vi "Initialize From Config.vi"(8 "error in":errorcluster, 9 "Modules":refnum<class "TBM module execution interface.lvclass">[](array[class]), 10 "Module Configurations":refnum<class "TBM module configuration.lvclass">[](array[class]), 11 "Engine Configuration":refnum<class "Standard Engine Configuration.lvclass">) -> (0 "error out":errorcluster, 3 "Engine Data Out":T1={"timed loop timer source"={"Processor"=-2, "Priority"=0, "timing source dt"=2, "timer source"=refnum}, "control loop data"={"engine tag bus"={"Double"=[], "Single"=[], "I64"=[], "I32"=[], "I16"=[], "I8"=[], "U64"=[], "U32"=[], "U16"=[], "U8"=[], "Boolean"=[], "String"=[], "Array of Double"=[], "Array of Single"=[], "Array of I64"=[], "Array of I32"=[], "Array of I16"=[], "Array of I8"=[], "Array of U64"=[], "Array of U32"=[], "Array of U16"=[], "Array of U8"=[], "Array of Boolean"=[], "Array of String"=[]}, "engine schedule"={"module run flags"=[], "decimation schedule"={"decimations"=[], "offsets"=[]}}, "module information"=[]}, "status reporting"={"late? index (bool)"=-1, "late count index (U32)"=-1, "dt (ns) index (U64)"=-1, "execution time (ns) index (U64)"=-1}})   [LabVIEW 2013, in "Standard Engine Runtime.lvclass"]
doc: "This VI contains all of the logic necessary for configuring the engine based on a given engine configuration, and an array of modules with their configurations. \n\nFirst it allows the modules to finish configuring themselves by calling their dynamic configuration and mapping functions. \n\nThen it calls the Init method for each module and initializes their channel data space as well as the engine's tag data space. \n\nIt also initializes all of the other features of the engine including the timing source, decimation, error handling, execution order, etc."
uses:
  Standard Engine Runtime.lvclass
  main engine/Engine Data.ctl
  <vilib>/NI/Module Timing Source/timing source/TBM timing source.lvclass
  main engine/timed loop timing sources.ctl
  main engine/control loop data.ctl
  <vilib>/NI/Tag Bus/table/data table.ctl
  main engine/engine run schedule.ctl
  main engine/engine decimation schedule.ctl
  main engine/full module data.ctl
  <vilib>/NI/Tag Bus Module Framework/runtime/TBM module execution interface.lvclass
  main engine/module run state.ctl
  async executor/asynchronous executor reference.ctl
  async executor/async message to executor.ctl
  async command notification.ctl
  async error info.ctl
  <vilib>/NI/Tag Bus Module Framework/runtime/error classification.ctl
  <vilib>/NI/Tag Bus Module Framework/module configuration/TBM module configuration.lvclass
  main engine/module method data.ctl
  <vilib>/NI/Tag Bus/table/transfer specification.ctl
  <vilib>/NI/Tag Bus/tag/Data Type.ctl
  main engine/fault handling spec.ctl
  Configuration/Error Actions.ctl
  main engine/status reporting data.ctl
  Configuration/Standard Engine Configuration.lvclass
  Configuration/Standard Engine Configuration.lvclass/Standard Engine Configuration.ctl
  <vilib>/NI/Configuration Framework/serializable configuration/NISE_CEF_serializable configuration.lvclass/NISE_CEF_serializable configuration.ctl
  <vilib>/NI/Module Timing Source/standard timing source/ms timing source.lvclass
  <vilib>/NI/Module Timing Source/usec timing source/usec timing source.lvclass
  <vilib>/NI/Module Timing Source/scan engine timing source/scan engine timing source.lvclass
  <vilib>/NI/Module Execution Interface/Engine Configuration/engine configuration.lvclass/engine configuration.ctl
  <vilib>/NI/Tag Bus/dictionary/data dictionary.lvclass/data dictionary.ctl
  <vilib>/NI/Tag Bus/dictionary/lookup polymorphs/locate double.vi
  <vilib>/NI/Tag Bus/dictionary/lookup polymorphs/locate I32.vi
  Configuration/Read Processor.vi
  Configuration/Read Priority.vi
  Configuration/Read Master Timing Module.vi
  Configuration/Read Timing Source Type.vi
  Configuration/Read enable module timing info.vi
  <vilib>/NI/Tag Bus/dictionary/search/find data index.vi
  <vilib>/NI/Tag Bus/dictionary/search/search string list.vi
  Configuration/Read Timing Source dt.vi
  <vilib>/Utility/LVClass/Get LV Class Name.vi
  <vilib>/NI/Configuration Framework/error generator/NISE_error generator.vi
  Configuration/Find Module Specific Config.vi
  <vilib>/NI/Configuration Framework/serializable configuration/get alias.vi
  <vilib>/NI/Tag Bus/dictionary/tag not found.vi
  <vilib>/Utility/RT CPU pool selections.ctl
  <vilib>/NI/Tag Bus/dictionary/data dictionary.lvclass
  <vilib>/NI/Module Execution Interface/Engine Configuration/engine configuration.lvclass
  <vilib>/NI/Module Execution Interface/Engine Runtime/Engine Runtime Interface.lvclass
  main engine/main engine.lvlib
  <vilib>/NI/Configuration Framework/serializable configuration/NISE_CEF_serializable configuration.lvclass
  <vilib>/NI/Tag Bus/table/data table.lvlib
  <vilib>/NI/Tag Bus/tag/tag descriptor.lvclass
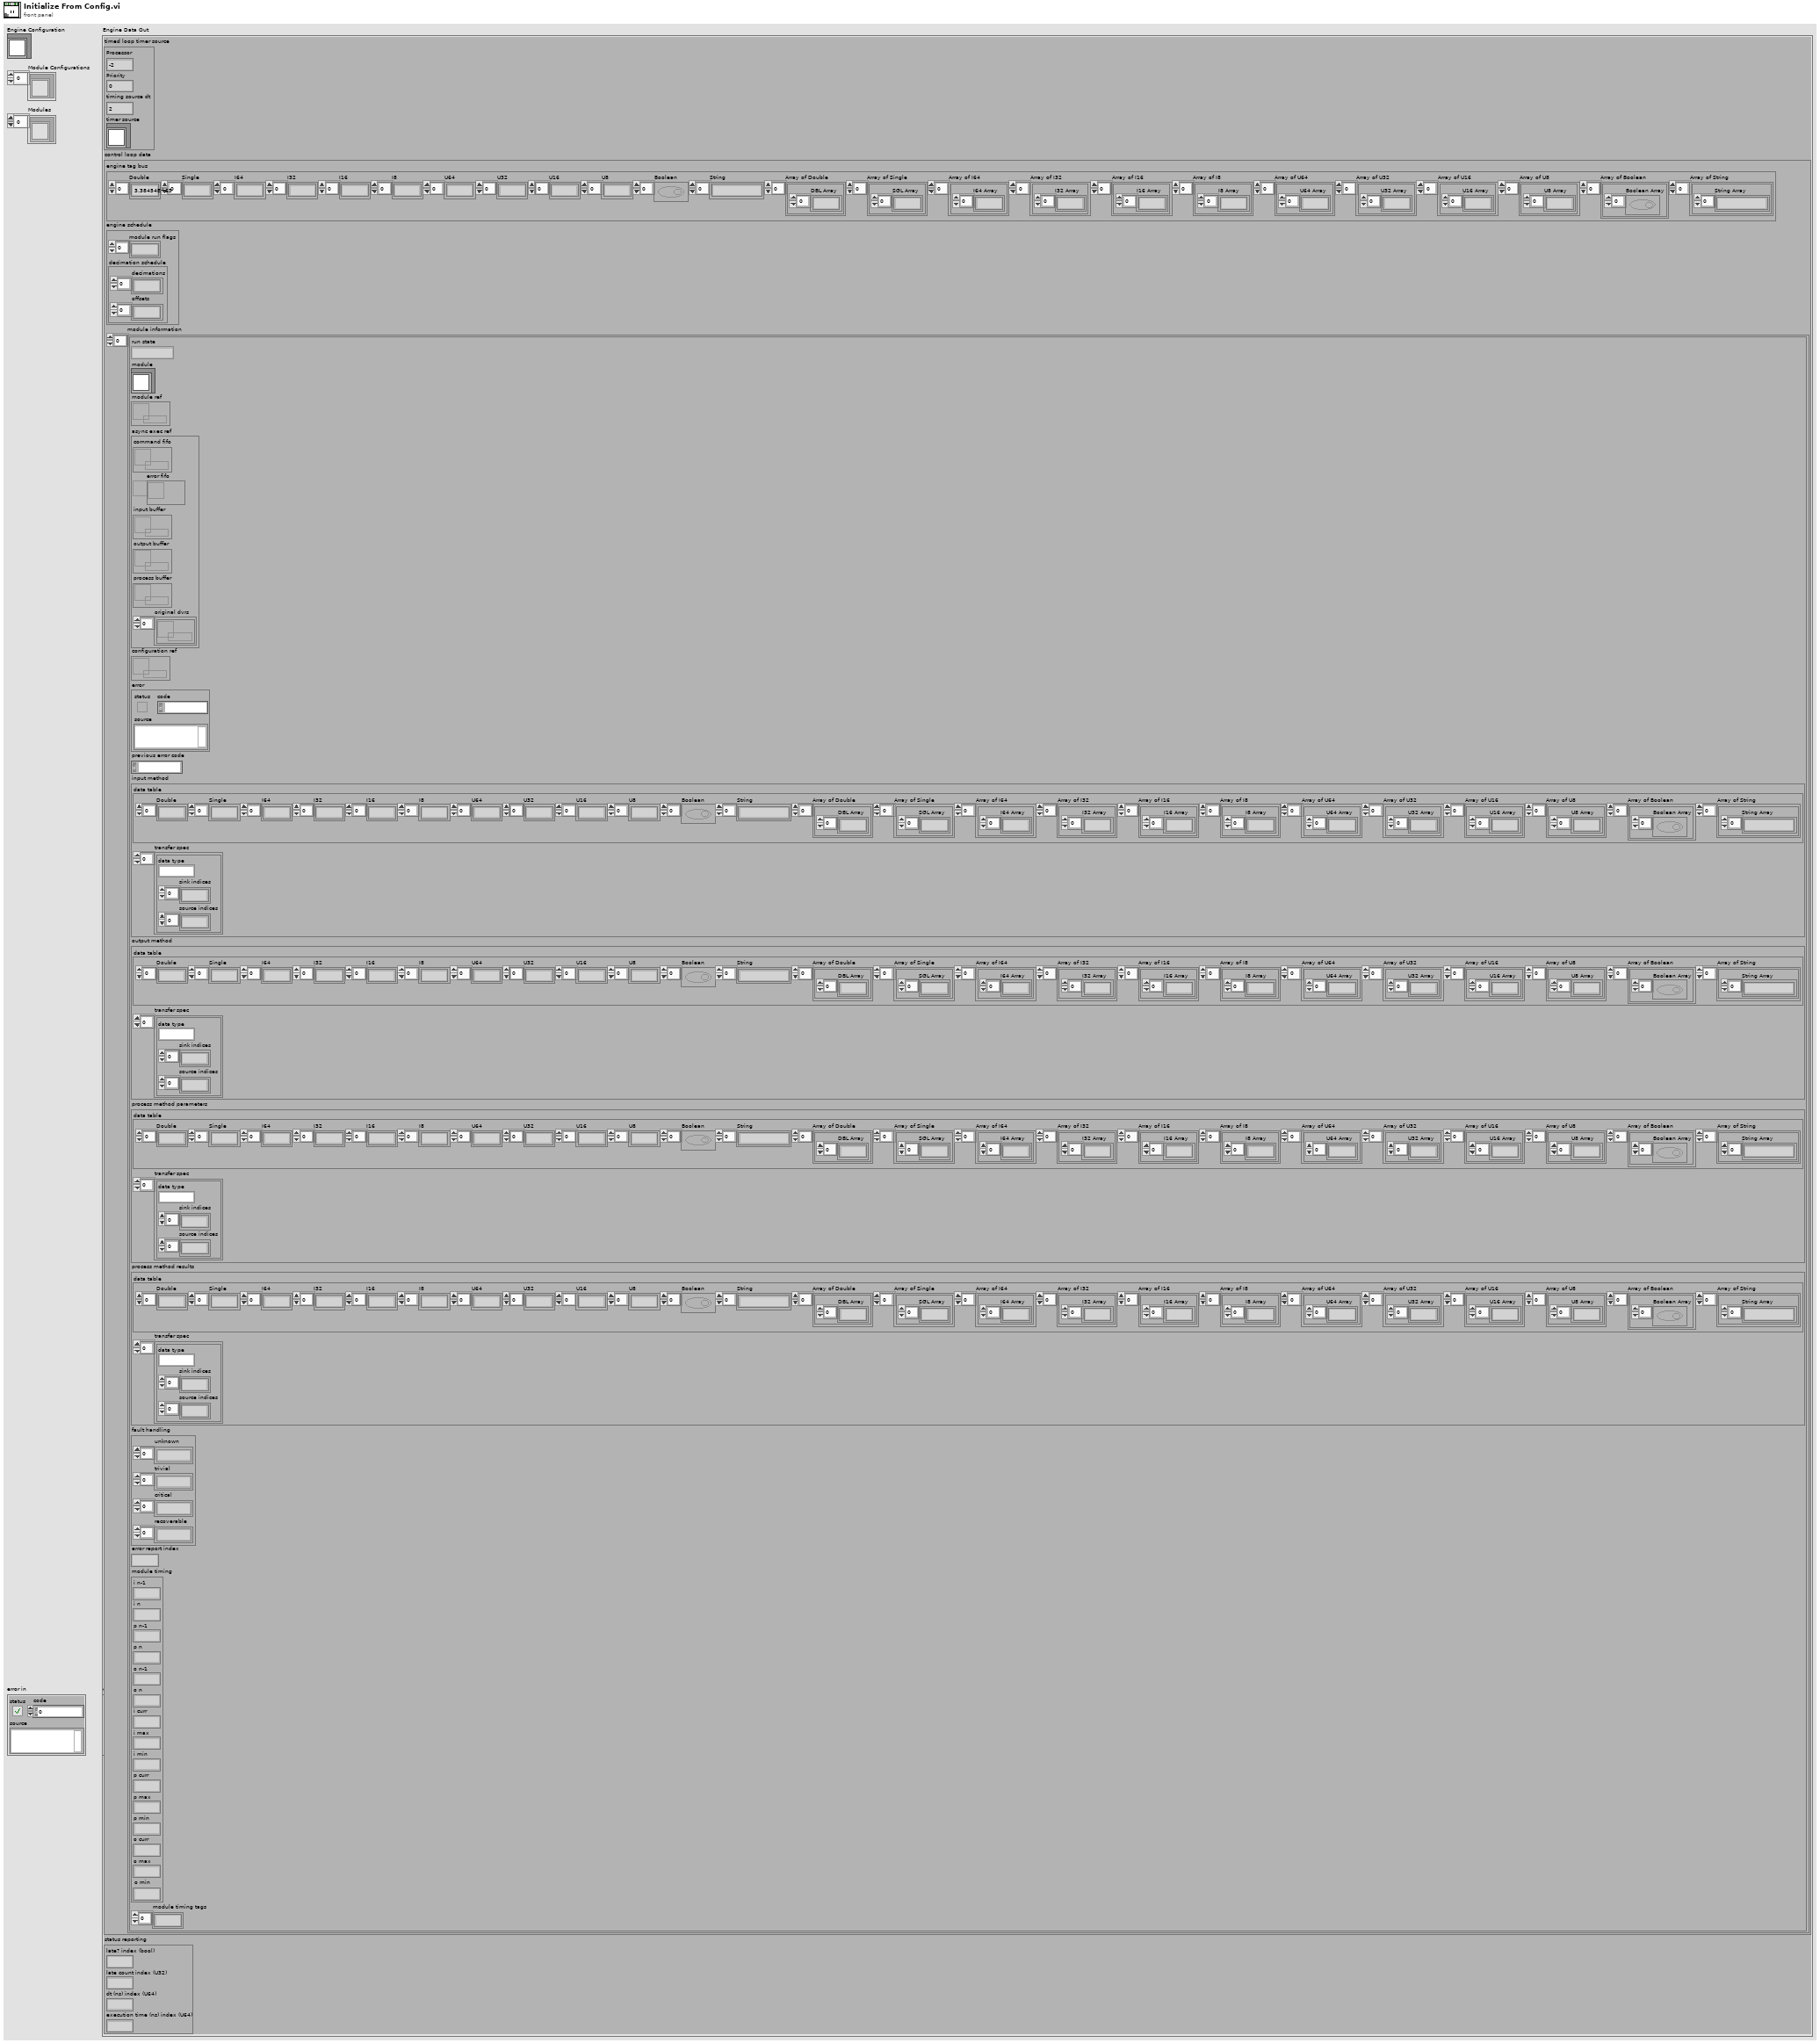
[diagram p1: front panel]
types:
  T1 = typedef "main engine.lvlib/Engine Data.ctl" = cluster{"timed loop timer source":T2, "control loop data":T3, "status reporting":T15}
  T2 = typedef "main engine.lvlib/timed loop timing sources.ctl" = cluster{"Processor":i32, "Priority":i32, "timing source dt":u32, "timer source":refnum<class "TBM timing source.lvclass">}
  T3 = typedef "main engine.lvlib/control loop data.ctl" = cluster{"engine tag bus":T4, "engine schedule":T5, "module information":T7[]}
  T4 = typedef "tag bus.lvlib/data table.lvlib/data table.ctl" = cluster{"Double":dbl[], "Single":sgl[], "I64":i64[], "I32":i32[], "I16":i16[], "I8":i8[], "U64":u64[], "U32":u32[], "U16":u16[], "U8":u8[], "Boolean":bool[], "String":string[], "Array of Double":cluster{"DBL Array":dbl[]}[], "Array of Single":cluster{"SGL Array":sgl[]}[], "Array of I64":cluster{"I64 Array":i64[]}[], "Array of I32":cluster{"I32 Array":i32[]}[], "Array of I16":cluster{"I16 Array":i16[]}[], "Array of I8":cluster{"I8 Array":i8[]}[], "Array of U64":cluster{"U64 Array":u64[]}[], "Array of U32":cluster{"U32 Array":u32[]}[], "Array of U16":cluster{"U16 Array":u16[]}[], "Array of U8":cluster{"U8 Array":u8[]}[], "Array of Boolean":cluster{"Boolean Array":bool[]}[], "Array of String":cluster{"String Array":string[]}[]}
  T5 = typedef "main engine.lvlib/engine run schedule.ctl" = cluster{"module run flags":u8[], "decimation schedule":T6}
  T6 = typedef "main engine.lvlib/engine decimation schedule.ctl" = cluster{"decimations":u16[], "offsets":u16[]}
  T7 = typedef "main engine.lvlib/full module data.ctl" = cluster{"run state":T8, "module":refnum<class "TBM module execution interface.lvclass">, "module ref":refnum<data-value>, "async exec ref":T9, "configuration ref":refnum<data-value>, "error":errorcluster, "previous error code":i32, "input method":T10, "output method":T10, "process method parameters":T10, "process method results":T10, "fault handling":T13, "error report index ":i32, "module timing":cluster{"i n-1":dbl, "i n":dbl, "p n-1":dbl, "p n":dbl, "o n-1":dbl, "o n":dbl, "i curr":dbl, "i max":dbl, "i min":dbl, "p curr":dbl, "p max":dbl, "p min":dbl, "o curr":dbl, "o max":dbl, "o min":dbl}, "module timing tags":i32[]}
  T8 = typedef "main engine.lvlib/module run state.ctl" = enum16{"sync", "async"}
  T9 = typedef "main engine.lvlib/asynchronous executor reference.ctl" = cluster{"command fifo":refnum<k33>, "error fifo":refnum<k33>, "input buffer":refnum<k33>, "output buffer":refnum<k33>, "process buffer":refnum<k33>, "original dvrs":refnum<data-value>[]}
  T10 = typedef "main engine.lvlib/module method data.ctl" = cluster{"data table":T4, "transfer spec":T11[]}
  T11 = typedef "tag bus.lvlib/data table.lvlib/transfer specification.ctl" = cluster{"data type":T12, "sink indices":i32[], "source indices":i32[]}
  T12 = typedef "tag bus.lvlib/tag descriptor.lvclass/Data Type.ctl" = enum16{"Double", "Single", "I64", "I32", "I16", "I8", "U64", "U32", "U16", "U8", "Boolean", "String", "Array of Double", "Array of Single", "Array of I64", "Array of I32", "Array of I16", "Array of I8", "Array of U64", "Array of U32", "Array of U16", "Array of U8", "Array of Boolean", "Array of String"}
  T13 = typedef "main engine.lvlib/fault handling spec.ctl" = cluster{"unknown":T14[], "trivial":T14[], "critical":T14[], "recoverable":T14[]}
  T14 = typedef "Standard Engine Configuration.lvclass/Error Actions.ctl" = enum16{"Clear", "Notify", "Stop Component", "Stop Engine", "Safe State", "Attempt Recovery"}
  T15 = typedef "main engine.lvlib/status reporting data.ctl" = cluster{"late? index (bool)":i32, "late count index (U32)":i32, "dt (ns) index (U64)":i32, "execution time (ns) index (U64)":i32}
  T16 = typedef "Standard Engine Configuration.lvclass/Supported Timing Sources.ctl" = enum16{"Use Module Timing Source", "1 kHz Clock", "1 MHz Clock", "Synchronize to Scan Engine"}
  T17 = cluster{"execution order priority":i32, "Component Runtime Interface.lvclass":refnum<class "TBM module execution interface.lvclass">, "configuration out":refnum<class "TBM module configuration.lvclass">}
  T18 = cluster{"execution order priority":i32, "Component Runtime Interface.lvclass":refnum<class "TBM module execution interface.lvclass">, "configuration out":refnum<class "TBM module configuration.lvclass">}[]
  T19 = typedef "TBM channel.lvclass/data tables.ctl" = cluster{"input data":T20, "processing parameter":T20, "processing result":T20, "output data":T20}
  T20 = typedef "tag bus.lvlib/dictionary table pair.ctl" = cluster{"data dictionary":refnum<class "data dictionary.lvclass">, "data table":T4}
  T21 = typedef "TBM module execution interface.lvclass/execution settings.ctl" = cluster{"reads inputs":bool, "processes data":bool, "writes outputs":bool}
  T22 = typedef "Standard Engine Configuration.lvclass/error responses.ctl" = cluster{"unknown":T23, "trivial":T23, "critical":T23, "recoverable":T23}
  T23 = typedef "Standard Engine Configuration.lvclass/error options.ctl" = cluster{"clear":bool, "notify":bool, "remove module":bool, "abort engine":bool, "go to safe state":bool, "recover module":bool}
  T24 = typedef "Standard Engine Configuration.lvclass/Module Decimation.ctl" = cluster{"Decimation":u16, "Offset":u16, "sort order":i32, "async?":bool}
  T25 = typedef "Standard Engine Configuration.lvclass/timing reporting tags.ctl" = cluster{"late index (bool)":string, "late count index (U32)":string, "current dt ns(U64)":string, "last exec time ns(U64)":string}
  T26 = typedef "NI_Real-Time Target Support.lvlib/RT CPU pool selections.ctl" = enum16{"System & Timed Structures", "System", "Timed Structures", "Reserved"}
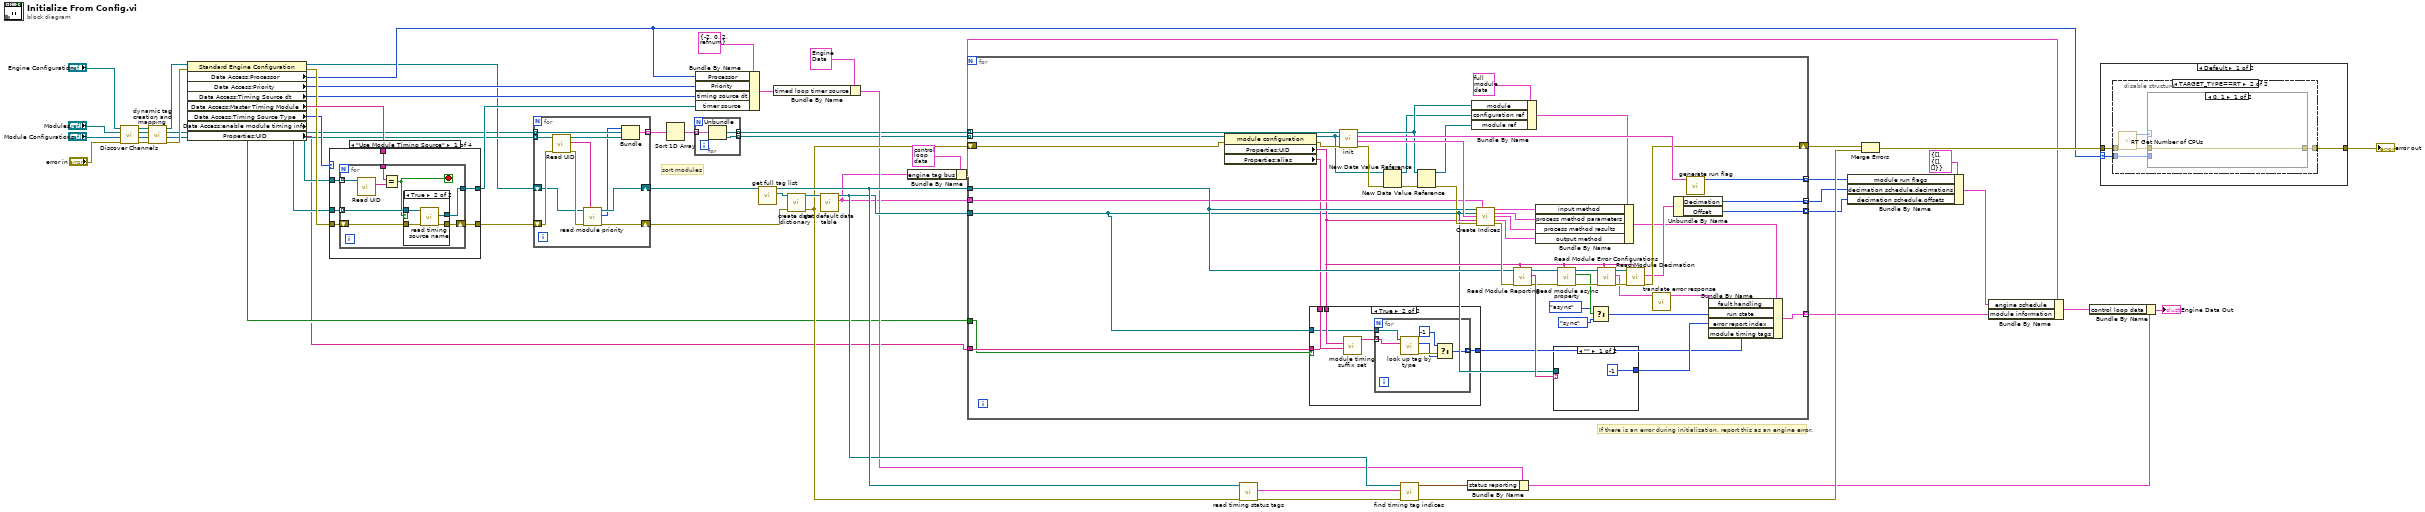
[diagram p0: block diagram]
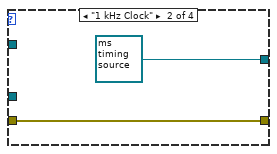
[diagram p3: hidden frame]
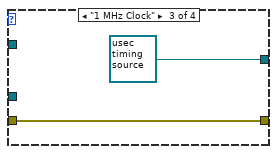
[diagram p4: hidden frame]
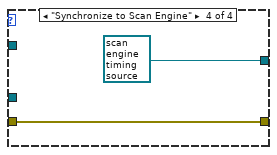
[diagram p5: hidden frame]
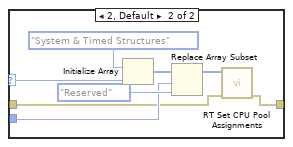
[diagram p7: hidden frame]
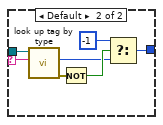
[diagram p10: hidden frame]
diagram:
  # "sort modules"
  # "If there is an error during initialization, report this as an engine error."
  n1 = call <vilib>:"Discover Channels.vi"("error in (no error)"="error in", "module configurations"="Module Configurations", "modules"="Modules", "engine configuration"="Engine Configuration") -> ("error out"=w52:errorcluster, "module configurations out"=w53:refnum<class "TBM module configuration.lvclass">[], "modules out"=w54:refnum<class "TBM module execution interface.lvclass">[], "engine configuration out"=w55:refnum<class "Standard Engine Configuration.lvclass">)  [unwired: 4 in]
  n2 = call <vilib>:"dynamic tag creation and mapping.vi"("error in"=w52, "module configurations"=w53, "modules"=w54, "engine configuration in"=w55) -> ("error out"=w46:errorcluster, "module configurations out"=w17:refnum<class "TBM module configuration.lvclass">[], "modules out"=w14:refnum<class "TBM module execution interface.lvclass">[], "engine configuration out"=w47:refnum<class "Standard Engine Configuration.lvclass">)  [unwired: 4 in]
  n3 = property class="Standard Engine Configuration"(reference=w47, error in=w46) -> (reference out=w16:refnum<class "Standard Engine Configuration.lvclass">, error out=w41:errorcluster, "Data Access:Processor"=w31:i32, "Data Access:Priority"=w30:i32, "Data Access:Timing Source dt"=w29:u32, "Data Access:Master Timing Module"=w42:string, "Data Access:Timing Source Type"=w32:T16, "Data Access:enable module timing info"=w2:bool, "Properties:UID"=w1:string)
  n4 = case shown="\"Use Module Timing Source\"" w32 {
    tunnel: [w60 refnum<class "ms timing source.lvclass"> refnum ("ms timing source.lvclass") refnum<class "usec timing source.lvclass"> refnum ("usec timing source.lvclass") refnum<class "scan engine timing source.lvclass"> refnum ("scan engine timing source.lvclass")] -> w40
    tunnel: w17 -> [w63 _ _ _]
    tunnel: w14 -> [w62 _ _ _]
    tunnel: w42 -> [w61 _ _ _]
    tunnel: [w59 w77 w79 w81] -> w13
    tunnel: w41 -> [w58 w77 w79 w81]
    frame "Use Module Timing Source" {
      n5 = for {
        tunnel: w63 -> [w71] mode=indexing
        tunnel: w62 -> [w68] mode=indexing
        tunnel: w61 -> [w69]
        tunnel: [w66] -> w60
        shift-right: [w65] -> w59
        shift-left: w58 -> [w64]
        stop <- w67 stop-if-true
        n6 = call <vilib>:"Read UID.vi"("configuration in"=w71) -> ("instance id"=w70:string)  [unwired: 8 in, 2 out]
        n7 = Equal?(x=w69, y=w70) -> (x = y?=w67:bool)
        n8 = case shown="True" w67 {
          tunnel: w68 -> [_ w76]
          tunnel: [_ w75] -> w66
          tunnel: [w72 w74] -> w65
          tunnel: w64 -> [w72 w73]
          frame False {
          }
          frame True {
            n9 = call-dynamic "read timing source name.vi"("error in"=w73, "module in"=w76) -> ("error out"=w74:errorcluster, "timing source"=w75:refnum<class "TBM timing source.lvclass">)  [unwired: 7 in, 1 out]
          }
        }
      }
    }
    frame "1 kHz Clock" {
    }
    frame "1 MHz Clock" {
    }
    frame "Synchronize to Scan Engine" {
    }
  }
  n10 = for {
    tunnel: w17 -> [w93] mode=indexing
    shift-right: [w89] -> w15
    shift-left: w16 -> [w87]
    tunnel: w14 -> [w86] mode=indexing
    shift-right: [w92] -> w12
    shift-left: w13 -> [w91]
    tunnel: [w83] -> w11 mode=indexing
    n11 = call <vilib>:"Read UID.vi"("error in"=w91, "configuration in"=w93) -> ("error out"=w90:errorcluster, "instance id"=w88:string, "configuration out"=w85:refnum<class "TBM module configuration.lvclass">)  [unwired: 7 in]
    n12 = call "read module priority.vi"("Module ID"=w88, "error in"=w90, "Standard Engine Repo Data in"=w87) -> ("error out"=w92:errorcluster, "execution order priority"=w84:i32, "Standard Engine Repo Data out"=w89:refnum<class "Standard Engine Configuration.lvclass">)  [unwired: 6 in]
    n13 = Bundle("execution order priority"=w84, "Component Runtime Interface.lvclass"=w86, "configuration out"=w85) -> (w83:T17)  [unwired: 1 in]
  }
  n14 = Sort 1D Array(array=w11) -> (sorted array=w10:T18)
  n15 = for {
    tunnel: w10 -> [w96] mode=indexing
    tunnel: [w95] -> w9 mode=indexing
    tunnel: [w94] -> w8 mode=indexing
    n16 = Unbundle(w96) -> ("Component Runtime Interface.lvclass"=w95:refnum<class "TBM module execution interface.lvclass">, "configuration out"=w94:refnum<class "TBM module configuration.lvclass">)  [unwired: 1 out]
  }
  n17 = Bundle By Name(cluster=T2 {"Processor"=-2, "Priority"=0, "timing source dt"=2, "timer source"=refnum} ("timed loop timer source"), "Processor"=w31, "Priority"=w30, "timing source dt"=w29, "timer source"=w40) -> (w27:T2)
  n18 = call <vilib>:"get full tag list.vi"("engine configuration in"=w15) -> ("tag list"=w45:refnum<class "tag descriptor.lvclass">[], "engine configuration out"=w39:refnum<class "Standard Engine Configuration.lvclass">)  [unwired: 9 in]
  n19 = Bundle By Name(cluster=T1 {"timed loop timer source"={"Processor"=-2, "Priority"=0, "timing source dt"=2, "timer source"=refnum}, "control loop data"={"engine tag bus"={"Double"=[], "Single"=[], "I64"=[], "I32"=[], "I16"=[], "I8"=[], "U64"=[], "U32"=[], "U16"=[], "U8"=[], "Boolean"=[], "String"=[], "Array of Double"=[], "Array of Single"=[], "Array of I64"=[], "Array of I32"=[], "Array of I16"=[], "Array of I8"=[], "Array of U64"=[], "Array of U32"=[], "Array of U16"=[], "Array of U8"=[], "Array of Boolean"=[], "Array of String"=[]}, "engine schedule"={"module run flags"=[], "decimation schedule"={"decimations"=[], "offsets"=[]}}, "module information"=[]}, "status reporting"={"late? index (bool)"=-1, "late count index (U32)"=-1, "dt (ns) index (U64)"=-1, "execution time (ns) index (U64)"=0}} ("Engine Data Out"), "timed loop timer source"=w27) -> (w26:T1)
  n20 = call <vilib>:"create data dictionary.vi"("error in"=w12, "system tags"=w45) -> ("error out"=w38:errorcluster, "data dictionary"=w44:refnum<class "data dictionary.lvclass">)  [unwired: 8 in]
  n21 = call <vilib>:"get default data table.vi"("data dictionary in"=w44) -> ("default data table"=w3:T4, "data dictionary out"=w35:refnum<class "data dictionary.lvclass">)  [unwired: 9 in]
  n22 = Bundle By Name(cluster=T3 {"engine tag bus"={"Double"=[], "Single"=[], "I64"=[], "I32"=[], "I16"=[], "I8"=[], "U64"=[], "U32"=[], "U16"=[], "U8"=[], "Boolean"=[], "String"=[], "Array of Double"=[], "Array of Single"=[], "Array of I64"=[], "Array of I32"=[], "Array of I16"=[], "Array of I8"=[], "Array of U64"=[], "Array of U32"=[], "Array of U16"=[], "Array of U8"=[], "Array of Boolean"=[], "Array of String"=[]}, "engine schedule"={"module run flags"=[], "decimation schedule"={"decimations"=[], "offsets"=[]}}, "module information"=[]} ("control loop data"), "engine tag bus"=w3) -> (w21:T3)
  n23 = for {
    tunnel: w8 -> [w141] mode=indexing
    shift-right: [w137] -> w57
    shift-left: w38 -> [w140]
    tunnel: w9 -> [w145] mode=indexing
    tunnel: w35 -> [w99]
    tunnel: w39 -> [w133]
    tunnel: [w132] -> w7 mode=indexing
    tunnel: [w130] -> w6 mode=indexing
    tunnel: [w129] -> w5 mode=indexing
    tunnel: [w111] -> w4 mode=indexing
    tunnel: w3 -> [w103]
    tunnel: w2 -> [w97]
    tunnel: w1 -> [w100]
    n24 = property class="module configuration"(reference=w141, error in=w140) -> (reference out=w118:refnum<class "TBM module configuration.lvclass">, error out=w136:errorcluster, "Properties:UID"=w101:string, "Properties:alias"=w102:string)
    n25 = case shown="True" w97 {
      tunnel: w102 -> [_ w151]
      tunnel: w101 -> [_ w150]
      tunnel: w100 -> [_ w149]
      tunnel: w99 -> [_ w148]
      tunnel: [_ w146] -> w98
      frame False {
      }
      frame True {
        n26 = call "module timing suffix set.vi"("mod alias"=w151, "mod id"=w150, "eng id"=w149) -> ("names"=w147:string[])  [unwired: 8 in]
        n27 = for {
          tunnel: w148 -> [w157]
          tunnel: w147 -> [w156] mode=indexing
          tunnel: [w152] -> w146 mode=indexing
          n28 = call-poly <vilib>:"look up tag by type.vi"("name"=w156, "data dictionary in"=w157) -> ("error out"=w155:errorcluster, "index"=w154:i32)  [unwired: 7 in, 1 out]
          n29 = Select(t=-1, s=w155, f=w154) -> (s? t:f=w152:i32)
        }
      }
    }
    n30 = call-dynamic "init.vi"("error in"=w136, "module configuration"=w118, "module in"=w145) -> ("error out"=w144:errorcluster, "data allocations"=w142:T19, "execution settings"=w143:T21, "module out"=w116:refnum<class "TBM module execution interface.lvclass">)  [unwired: 5 in]
    n31 = New Data Value Reference(data value=w118, error in=w144) -> (data value reference=w115:refnum<data-value>, error out=w120:errorcluster)
    n32 = New Data Value Reference(data value=w116, error in=w120) -> (data value reference=w117:refnum<data-value>, error out=w119:errorcluster)
    n33 = Bundle By Name(cluster=T7 {"run state"=enum."sync", "module"=refnum, "module ref"=refnum, "async exec ref"={"command fifo"=refnum, "error fifo"=refnum, "input buffer"=refnum, "output buffer"=refnum, "process buffer"=refnum, "original dvrs"=[]}, "configuration ref"=refnum, "error"={"status"=FALSE, "code"=0, "source"=""}, "previous error code"=0, "input method"={"data table"={"Double"=[], "Single"=[], "I64"=[], "I32"=[], "I16"=[], "I8"=[], "U64"=[], "U32"=[], "U16"=[], "U8"=[], "Boolean"=[], "String"=[], "Array of Double"=[], "Array of Single"=[], "Array of I64"=[], "Array of I32"=[], "Array of I16"=[], "Array of I8"=[], "Array of U64"=[], "Array of U32"=[], "Array of U16"=[], "Array of U8"=[], "Array of Boolean"=[], "Array of String"=[]}, "transfer spec"=[]}, "output method"={"data table"={"Double"=[], "Single"=[], "I64"=[], "I32"=[], "I16"=[], "I8"=[], "U64"=[], "U32"=[], "U16"=[], "U8"=[], "Boolean"=[], "String"=[], "Array of Double"=[], "Array of Single"=[], "Array of I64"=[], "Array of I32"=[], "Array of I16"=[], "Array of I8"=[], "Array of U64"=[], "Array of U32"=[], "Array of U16"=[], "Array of U8"=[], "Array of Boolean"=[], "Array of String"=[]}, "transfer spec"=[]}, "process method parameters"={"data table"={"Double"=[], "Single"=[], "I64"=[], "I32"=[], "I16"=[], "I8"=[], "U64"=[], "U32"=[], "U16"=[], "U8"=[], "Boolean"=[], "String"=[], "Array of Double"=[], "Array of Single"=[], "Array of I64"=[], "Array of I32"=[], "Array of I16"=[], "Array of I8"=[], "Array of U64"=[], "Array of U32"=[], "Array of U16"=[], "Array of U8"=[], "Array of Boolean"=[], "Array of String"=[]}, "transfer spec"=[]}, "process method results"={"data table"={"Double"=[], "Single"=[], "I64"=[], "I32"=[], "I16"=[], "I8"=[], "U64"=[], "U32"=[], "U16"=[], "U8"=[], "Boolean"=[], "String"=[], "Array of Double"=[], "Array of Single"=[], "Array of I64"=[], "Array of I32"=[], "Array of I16"=[], "Array of I8"=[], "Array of U64"=[], "Array of U32"=[], "Array of U16"=[], "Array of U8"=[], "Array of Boolean"=[], "Array of String"=[]}, "transfer spec"=[]}, "fault handling"={"unknown"=[], "trivial"=[], "critical"=[], "recoverable"=[]}, "error report index "=0, "module timing"={"i n-1"=0.0, "i n"=0.0, "p n-1"=0.0, "p n"=0.0, "o n-1"=0.0, "o n"=0.0, "i curr"=0.0, "i max"=0.0, "i min"=0.0, "p curr"=0.0, "p max"=0.0, "p min"=0.0, "o curr"=0.0, "o max"=0.0, "o min"=0.0}, "module timing tags"=[]} ("module data"), "module"=w116, "configuration ref"=w115, "module ref"=w117) -> (w112:T7)
    n34 = call "Create Indices.vi"("Standard Engine Configuration"=w133, "Engine Tags"=w103, "main data dictionary"=w99, "data description"=w142, "Module ID"=w101, "error in"=w119) -> ("Input Transfer Specification"=w110:T10, "Parameter Transfer Specifcation"=w109:T10, "Result Transfer Specifcation"=w108:T10, "Output Transfer Specifcation"=w107:T10, "error out"=w135:errorcluster)  [unwired: 5 in]
    n35 = call "Read Module Reporting.vi"("Module ID"=w101, "error in"=w135, "Standard Engine Repo Data in"=w133) -> ("error out"=w126:errorcluster, "error tag"=w134:string, "Standard Engine Repo Data out"=w127:refnum<class "Standard Engine Configuration.lvclass">)  [unwired: 6 in]
    n36 = Bundle By Name(cluster=w112, "input method"=w110, "process method parameters"=w109, "process method results"=w108, "output method"=w107) -> (w113:T7)
    n37 = case shown="\"\"" w134 {
      selector: w134 -> [_ w163]
      tunnel: w99 -> [_ w165]
      tunnel: [-1 ("index") w159] -> w106
      frame "" {
      }
      frame Default {
        n38 = call-poly <vilib>:"look up tag by type.vi"("name"=w163, "data dictionary in"=w165) -> ("error out"=w164:errorcluster, "index"=w161:i32)  [unwired: 7 in, 1 out]
        n39 = Not(x=w164) -> (.not. x?=w162:bool)
        n40 = Select(t=-1 ("index"), s=w162, f=w161) -> (s? t:f=w159:i32)
      }
    }
    n41 = call "Read module async property.vi"("Module ID"=w101, "error in"=w126, "Standard Engine Repo Data in"=w127) -> ("error out"=w125:errorcluster, "async?"=w123:bool, "Standard Engine Repo Data out"=w124:refnum<class "Standard Engine Configuration.lvclass">)  [unwired: 6 in]
    n42 = Select(t=module_run_state."async" ("run state"), s=w123, f=module_run_state."sync" ("run state")) -> (s? t:f=w114:T8)
    n43 = call "Read Module Error Configurations.vi"("Module ID"=w101, "error in"=w125, "Standard Engine Repo Data in"=w124) -> ("error out"=w138:errorcluster, "error responses"=w104:T22, "Standard Engine Repo Data out"=w139:refnum<class "Standard Engine Configuration.lvclass">)  [unwired: 6 in]
    n44 = call "Read Module Decimation.vi"("Module ID"=w101, "error in"=w138, "Standard Engine Repo Data in"=w139) -> ("error out"=w137:errorcluster, "Module Decimation"=w131:T24)  [unwired: 6 in, 1 out]
    n45 = call "translate error response.vi"("error responses"=w104) -> ("fault handling"=w105:T13)  [unwired: 10 in]
    n46 = Unbundle By Name(w131) -> ("Decimation"=w130:u16, "Offset"=w129:u16)
    n47 = call "generate run flag.vi"("execution settings"=w143) -> ("run flags"=w132:u8)  [unwired: 10 in]
    n48 = Bundle By Name(cluster=w113, "fault handling"=w105, "run state"=w114, "error report index"=w106, "module timing tags"=w98) -> (w111:T7)
  }
  n49 = call "read timing status tags.vi"("error in"=w38, "Standard Engine Configuration in"=w39) -> ("error out"=w36:errorcluster, "timing reporting"=w37:T25)  [unwired: 7 in, 1 out]
  n50 = call "find timing tag indices.vi"("error in"=w36, "timing reporting"=w37, "data dictionary in"=w35) -> ("error out"=w34:errorcluster, "reporting indices"=w25:T15)  [unwired: 7 in]
  n51 = Bundle By Name(cluster=w26, "status reporting"=w25) -> (w24:T1)
  n52 = Bundle By Name(cluster=T5 {"module run flags"=[], "decimation schedule"={"decimations"=[], "offsets"=[]}} ("engine schedule"), "module run flags"=w7, "decimation schedule.decimations"=w6, "decimation schedule.offsets"=w5) -> (w18:T5)
  n53 = Merge Errors(w57, w34) -> (w43:errorcluster)
  n54 = Bundle By Name(cluster=w21, "engine schedule"=w18, "module information"=w4) -> (w20:T3)
  n55 = Bundle By Name(cluster=w24, "control loop data"=w20) -> (→"Engine Data Out":T1)
  n56 = case shown="Default" w31 {
    selector: w31 -> [w166 _]
    tunnel: w43 -> [w168 w184]
    tunnel: [w167 w184] -> w56
    frame Default {
      n57 = disable-structure shown="TARGET_TYPE==RT" {
        disable-tunnel: w168 -> [w169 w173]
        disable-tunnel: w166 -> [_ w171]
        disable-tunnel: [w169 w170] -> w167
        frame condition #0 (active) {
        }
        frame condition #1 {
          n58 = call <vilib>:"RT Get Number of CPUs.vi"("error in (no error)"=w173) -> ("error out"=w172:errorcluster, "# of CPUs"=w174:u32)  [unwired: 9 in]
          n59 = case shown="0, 1" w174 {
            selector: w174 -> [_ w182]
            tunnel: w172 -> [w175 w177]
            tunnel: w171 -> [_ w179]
            tunnel: [w175 w176] -> w170
            frame 0, 1 {
            }
            frame 2, Default {
              n60 = Initialize Array(RT_CPU_pool_selections."System & Timed Structures" ("Enum"), w182) -> (w181:T26[])
              n61 = Replace Array Subset(array=w181, new element=RT_CPU_pool_selections."Reserved" ("new element/subarray"), index=w179) -> (w178:T26[])
              n62 = call <vilib>:"RT Set CPU Pool Assignments.vi"("error in (no error)"=w177, "CPU pools"=w178) -> ("error out"=w176:errorcluster)  [unwired: 6 in, 3 out]
            }
          }
        }
      }
    }
    frame -2 {
    }
  }
  "error out" <- w56
